vi "Adaptive Transform (ADT) and Adaptive Expansion (ADE).vi"() -> ()   [LabVIEW 2023]
doc: "This example shows how to use the TFA Adaptive Transform VI and the TFA Adaptive Expansion VI.\n\n<b>Instructions:</b>\n1) Run this VI.\n2) Compare the original signal and reconstructed signal.\n3) Observe the values of the detected chirplets in the <b>Detected Chirplet by Adaptive Transform</b> section."
uses:
  <vilib>/addons/Time Frequency Analysis/Transform.llb/TFA Adaptive Transform (Waveform).vi
  <vilib>/addons/Time Frequency Analysis/Transform.llb/TFA Adaptive Expansion (Waveform).vi
  <vilib>/addons/_Advanced Signal Processing/NI_AdvSigProcTFA.lvlib
panel:
  out "aspt-left-top":bool
  in  "Data":u16(ring)=10 items=["PC Fan"=0, "Noisy Chirps"=1, "TDR 1"=2, "TDR 2"=3, "Liquefaction"=4, "Liquefaction Free"=5, "Aneurysm"=6, "Bat"=7, "RF"=8, "Two Gaussian"=9, "Three Gaussian"=10, "Chirp"=11, "Gaussian Chirp"=12, "Cross Chirp"=13, "Doppler"=14, "HOP"=15, "TF Sine"=16, "Three Tone"=17, "Four Tone"=23, "Blood Flow Doppler (phase a)"=20, "Blood Flow Doppler (phase b)"=21, "Heart sound"=22, "Random Noise"=19]
  out "Chirplet info":T1(array[cluster]) {"chirp rate" format="%#_2p Hz/s"; "frequency" format="%#_2p Hz"; "center" format="%#_2ps"; "standard deviation" format="%#_2ps"; "amplitude" format="%.2f"}
  out "Signals":waveform(dbl)[](graph)
  in  "Number of terms":i32=3
  # "Overview: Shows how to use the TFA Adaptive Transform VI and the TFA Adaptive Expansion VI.\nRequirements: LabVIEW Full Development System, Advanced Signal Processing Toolkit\nInstructions: \n1. Run this VI.\n2. Compare the original signal and reconstructed signal.\n3. Observe the values of the detected chirplets in the Detected Chirplet by Adaptive Transform section."
  # "Signal"
  # "Detected Chirplet by Adaptive Transform"
  # "Adaptive Transform Paras"
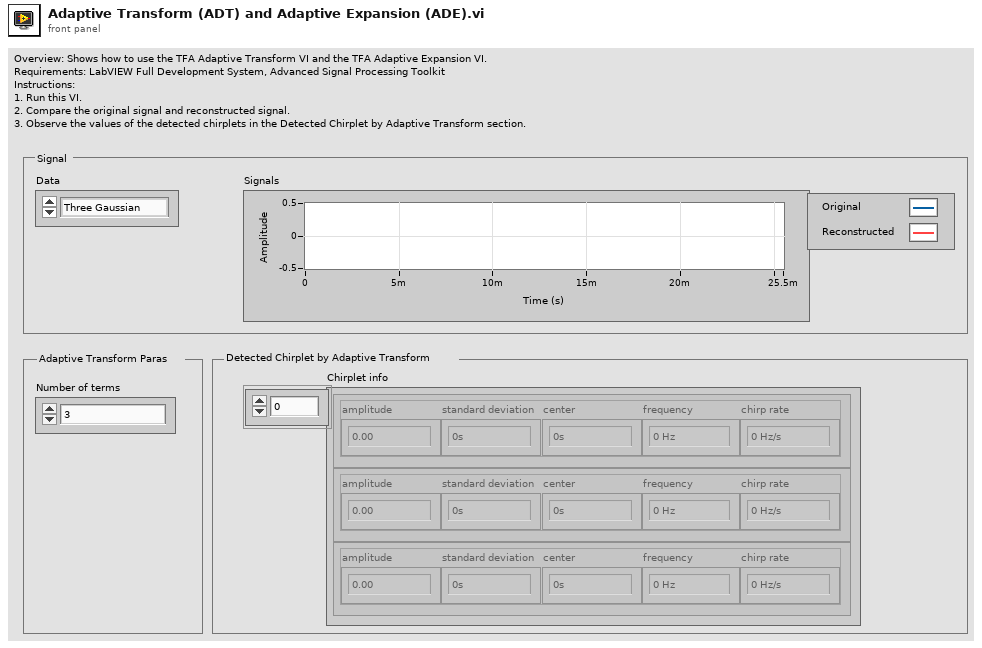
[diagram p1: front panel]
types:
  T1 = cluster{"amplitude":cdb, "standard deviation":dbl, "center":dbl, "frequency":dbl, "chirp rate":dbl}[]
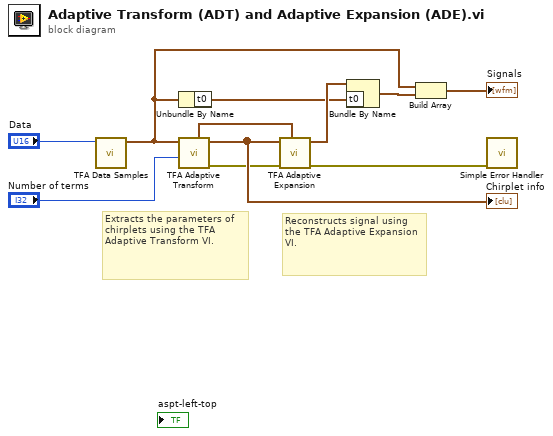
[diagram p0: block diagram]
diagram:
  # "Reconstructs signal using the TFA Adaptive Expansion VI."
  # "Extracts the parameters of chirplets using the TFA Adaptive Transform VI."
  n1 = call <vilib>:"TFA Data Samples.vi"("data"="Data") -> ("signal"=w8:waveform(dbl))  [unwired: 10 out]
  n2 = Unbundle By Name(w8) -> ("t0"=w3:timestamp)
  n3 = call-poly <vilib>:"TFA Adaptive Transform.vi"("number of terms"="Number of terms", "signal"=w8) -> ("error out"=w9:errorcluster, "chirplet info"=w11:T1, "sampling info"=w5:cluster{"sampling rate":dbl, "length":i32})  [unwired: 1 in, 6 out]
  "Chirplet info" <- w11
  n4 = call-poly <vilib>:"TFA Adaptive Expansion.vi"("sampling info"=w5, "error in (no error)"=w9, "chirplet info"=w11) -> ("error out"=w1:errorcluster, "signal"=w4:waveform(dbl))  [unwired: 1 in, 6 out]
  n5 = Bundle By Name(cluster=w4, "t0"=w3) -> (w2:waveform(dbl))
  n6 = Build Array(w8, w2) -> (→"Signals":waveform(dbl)[])
  n7 = call <vilib>:"Simple Error Handler.vi"("error in (no error)"=w1) -> ()  [unwired: 4 in, 5 out]
